vi "static background worker.vi"(11 "communicator in":refnum<class "communicator.lvclass">) -> ()   [LabVIEW 2015, in "communicator.lvclass"]
uses:
  communicator.lvclass
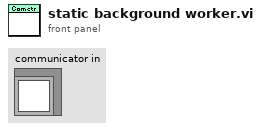
[diagram p1: front panel]
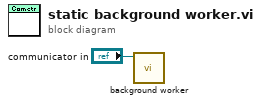
[diagram p0: block diagram]
diagram:
  n1 = call-dynamic "background worker.vi"("communicator in"="communicator in") -> ()  [unwired: 11 in]
